vi "Write STBD Motor.vi"(8 "error in (no error)":errorcluster, 10 "STBD Motor":T1, 11 "RDS State in":refnum<class "RDS State.lvclass">) -> (0 "error out":errorcluster, 3 "RDS State out":refnum<class "RDS State.lvclass">)   [LabVIEW 2015, in "RDS Child Messages.lvlib" / "RDS State.lvclass"]
uses:
  RDS State.lvclass
  Libraries/RDS Child Messages/MCB/MCB Motor Status.ctl
  RDS State.lvclass/RDS State.ctl
  Libraries/RDS Child Messages/RDS Child Messages.lvlib
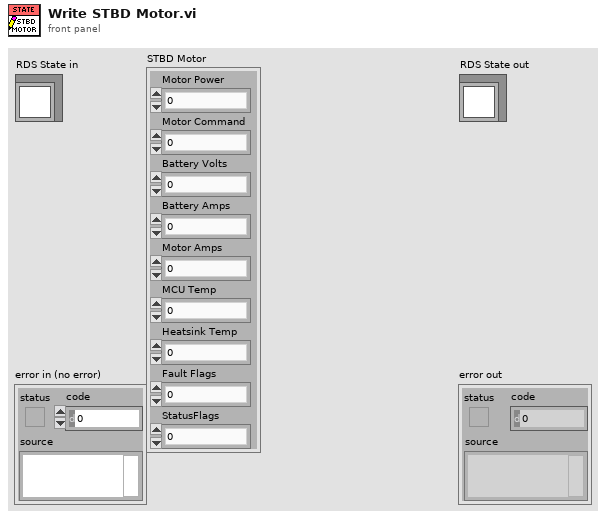
[diagram p1: front panel]
types:
  T1 = typedef "RDS Child Messages.lvlib/MCB Motor Status.ctl" = cluster{"Motor Power":i16, "Motor Command":i16, "Battery Volts":sgl, "Battery Amps":sgl, "Motor Amps":sgl, "MCU Temp":i16, "Heatsink Temp":i16, "Fault Flags":u16, "StatusFlags":u16}
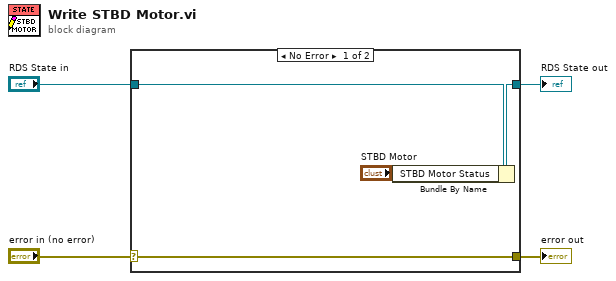
[diagram p0: block diagram]
diagram:
  n1 = case shown="No Error" "error in (no error)" {
    selector: "error in (no error)" -> [w8 w9]
    tunnel: [w8 w9] -> w3
    tunnel: [w6 w10] -> w1
    tunnel: "RDS State in" -> [w7 w10]
    frame No Error {
      n2 = Bundle By Name(cluster=w7, "STBD Motor Status"="STBD Motor") -> (w6:refnum<class "RDS State.lvclass">)
    }
    frame Error {
    }
  }
  "error out" <- w3
  "RDS State out" <- w1
